vi "Crossover v3.vi"(10 "Path In 2":T1={"Distance"=0.0, "Tour"=[1, 8, 6, 10, 4, 13, 16, 2, 3, 12, 15, 5, 9, 11, 14, 7, 1]}, 11 "Path In 1":T1={"Distance"=0.0, "Tour"=[1, 14, 13, 12, 7, 6, 15, 5, 11, 9, 10, 16, 3, 2, 4, 8, 1]}) -> (2 "Path Out 2":T1, 3 "Path Out 1":T1)   [LabVIEW 2015, in "TSP Library.lvlib"]
uses:
  TSP Library.lvlib
  TypeDef/Path.ctl
  <vilib>/Analysis/NI_AALBase.lvlib
panel:
  out "2 old":u16[](array[numeric])
  out "2 new":u16[](array[numeric])
  out "1 new":u16[](array[numeric])
  out "1 old":u16[](array[numeric])
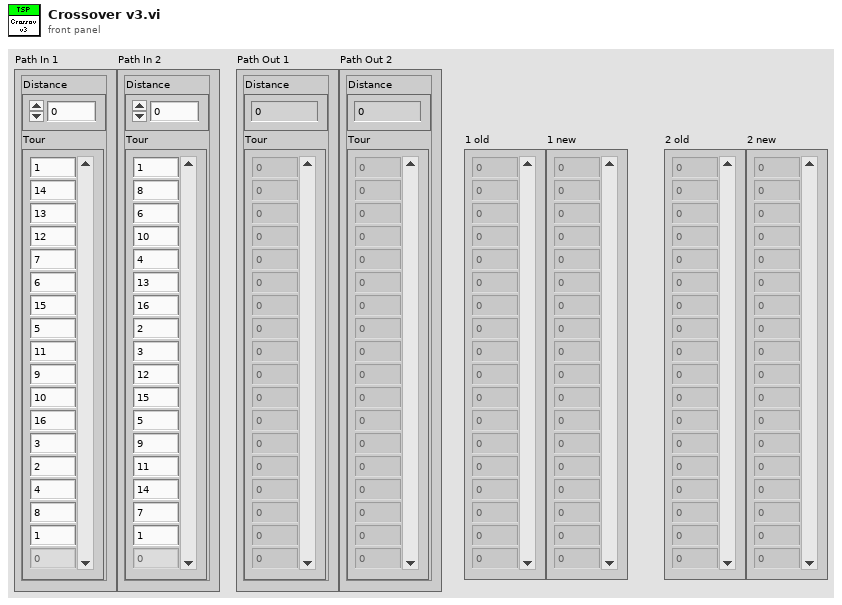
[diagram p1: front panel]
types:
  T1 = typedef "TSP Library.lvlib/Path.ctl" = cluster{"Distance":dbl, "Tour":u16[]}
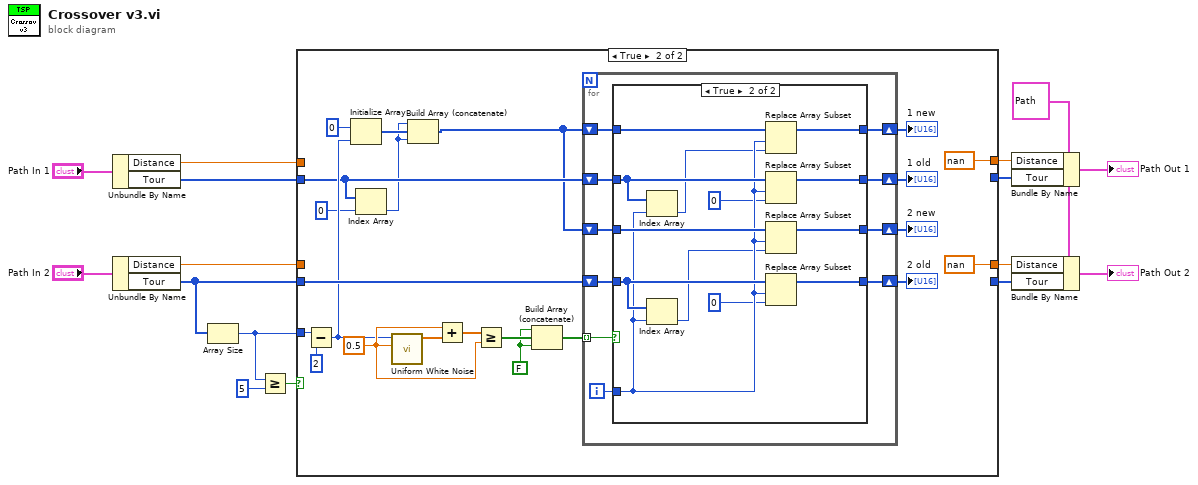
[diagram p0: block diagram]
diagram:
  w9 = T1 {"Distance"=0.0, "Tour"=[68, 82, 14, 66, 38, 76, 91, 89, 87, 84, 25, 25, 88]} ("Path In 1")
  n1 = Unbundle By Name("Path In 1") -> ("Distance"=w11:dbl, "Tour"=w12:u16[])
  n2 = Unbundle By Name("Path In 2") -> ("Distance"=w13:dbl, "Tour"=w14:u16[])
  n3 = Array Size(array=w14) -> (size(s)=w2:i32)
  n4 = Greater Or Equal?(x=w2, y=5) -> (x >= y?=w3:bool)
  n5 = case shown="True" w3 {
    tunnel: w2 -> [_ w42]
    tunnel: w14 -> [w17 w33]
    tunnel: w13 -> [w18 _]
    tunnel: w12 -> [w19 w29]
    tunnel: w11 -> [w20 _]
    tunnel: [w19 _] -> w7
    tunnel: [w17 _] -> w6
    tunnel: [w18 nan ("Distance")] -> w5
    tunnel: [w20 nan ("Distance")] -> w4
    frame False {
    }
    frame True {
      w34 = FALSE
      w36 = 0.5 ("amplitude")
      n6 = Subtract(x=w42, y=2) -> (x-y=w31:i32)
      n7 = Initialize Array(u16 0 ("Numeric"), w31) -> (w27:u16[])
      n8 = Index Array(array=w29, index=0) -> (element=w26:u16)
      n9 = call <vilib>:"Uniform White Noise.vi"("amplitude"=w36, "samples"=w31) -> ("uniform white noise"=w38:dbl[])  [unwired: 8 in, 1 out]
      n10 = Build Array (concatenate)(w26, w27, w26) -> (w25:u16[])
      n11 = Add(x=w36, y=w38) -> (x+y=w37:dbl[])
      n12 = Greater Or Equal?(x=w37, y=w36) -> (x >= y?=w35:bool[])
      n13 = Build Array (concatenate)(w34, w35, w34) -> (w32:bool[])
      n14 = for {
        tunnel: w32 -> [w52] mode=indexing
        shift-right: [w46] -> w22
        shift-left: w25 -> [w47]
        shift-right: [w50] -> w23
        shift-left: w25 -> [w51]
        shift-right: [w48] -> w24
        shift-left: w29 -> [w49]
        shift-right: [w44] -> w21
        shift-left: w33 -> [w45]
        i -> [w43]
        n15 = case shown="True" w52 {
          tunnel: [w56 w68] -> w50
          tunnel: w51 -> [w56 w69]
          tunnel: w49 -> [w55 w67]
          tunnel: [w55 w66] -> w48
          tunnel: w47 -> [w54 w65]
          tunnel: [w54 w64] -> w46
          tunnel: w45 -> [w53 w63]
          tunnel: [w53 w62] -> w44
          tunnel: w43 -> [_ w61]
          frame False {
          }
          frame True {
            n16 = Index Array(array=w67, index=w61) -> (element=w58:u16)
            n17 = Index Array(array=w63, index=w61) -> (element=w57:u16)
            n18 = Replace Array Subset(array=w69, new element=w58, index=w61) -> (w68:u16[])
            n19 = Replace Array Subset(array=w67, new element=u16 0 ("new element/subarray"), index=w61) -> (w66:u16[])
            n20 = Replace Array Subset(array=w65, new element=w57, index=w61) -> (w64:u16[])
            n21 = Replace Array Subset(array=w63, new element=u16 0 ("new element/subarray"), index=w61) -> (w62:u16[])
          }
        }
      }
      "1 old" <- w24
      "1 new" <- w23
      "2 new" <- w22
      "2 old" <- w21
    }
  }
  n22 = Bundle By Name(cluster=w9, "Distance"=w4, "Tour"=w7) -> (→"Path Out 1":T1)
  n23 = Bundle By Name(cluster=w9, "Distance"=w5, "Tour"=w6) -> (→"Path Out 2":T1)
